vi "Handle Error.vi"(8 "error in (no error)":errorcluster, 11 "NI in":refnum<class "NI.lvclass">) -> (0 "error out":errorcluster, 2 "stop actor?":bool=TRUE, 3 "NI out":refnum<class "NI.lvclass">)   [LabVIEW 2021, in "NI.lvlib" / "NI.lvclass"]
doc: "(<B>Filename</B>: Actor Framework.lvlib:Actor.lvclass:Handle Error.vi)\n\nDefines how the actor handles an error that occurred while processing a message. By default, this method does nothing except stop the actor."
uses:
  NI.lvclass
  <vilib>/ActorFramework/Actor/Actor.lvclass
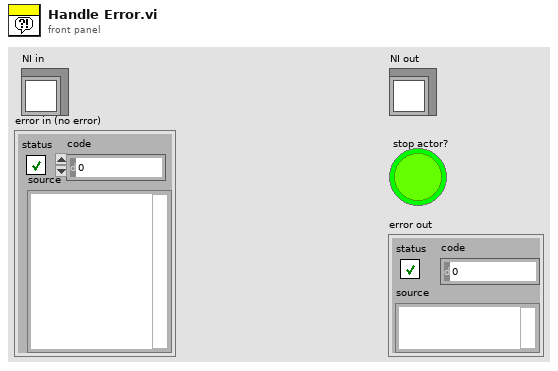
[diagram p1: front panel]
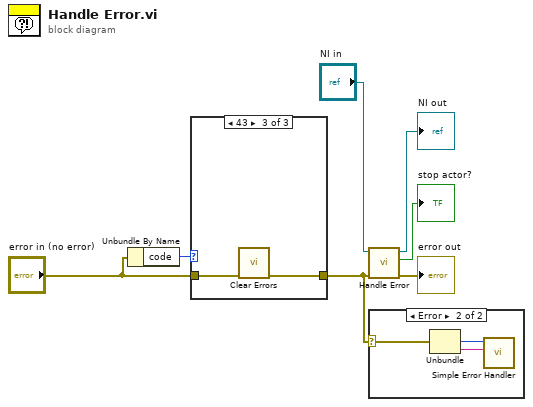
[diagram p0: block diagram]
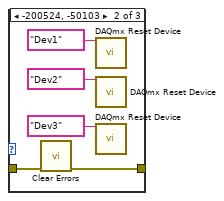
[diagram p4: hidden frame]
diagram:
  n1 = Unbundle By Name("error in (no error)") -> ("code"=w3:i32)
  n2 = case shown="43" w3 {
    tunnel: "error in (no error)" -> [w8 w10 w15]
    tunnel: [w8 w9 w14] -> w1
    frame Default {
    }
    frame -200524, -50103 {
      n3 = call <vilib>:"Clear Errors.vi"("error in (no error)"=w10) -> ("error out"=w9:errorcluster)  [unwired: 5 in, 1 out]
      n4 = call <vilib>:"DAQmx Reset Device.vi"("device in"=tag "Dev1") -> ()  [unwired: 14 in, 1 out]
      n5 = call <vilib>:"DAQmx Reset Device.vi"("device in"=tag "Dev2") -> ()  [unwired: 14 in, 1 out]
      n6 = call <vilib>:"DAQmx Reset Device.vi"("device in"=tag "Dev3") -> ()  [unwired: 14 in, 1 out]
    }
    frame 43 {
      n7 = call <vilib>:"Clear Errors.vi"("error in (no error)"=w15) -> ("error out"=w14:errorcluster)  [unwired: 5 in, 1 out]
    }
  }
  n8 = call-parent "Handle Error.vi"("error in (no error)"=w1, "Actor in"="NI in") -> ("error out"=→"error out":errorcluster, "stop actor?"=→"stop actor?":bool, "Actor out"=→"NI out":refnum<class "NI.lvclass">)  [unwired: 7 in]
  n9 = case shown="Error" w1 {
    selector: w1 -> [_ w18]
    frame No Error {
    }
    frame Error {
      n10 = Unbundle(w18) -> ("code"=w17:i32, "source"=w16:string)  [unwired: 1 out]
      n11 = call <vilib>:"Simple Error Handler.vi"("error code (no error:0)"=w17, "error source (\" \")"=w16) -> ()  [unwired: 3 in, 5 out]
    }
  }
